vi "NML data acq file names extract.vi"(0 "assign directory":bool, 1 "File name header":string="BaCrO_CCR", 3 "path in":path, 5 "From":string="12\n", 7 "To":string="2", 9 "Excluding From":string, 11 "Excluding To":string) -> (4 "path out":path, 6 "file paths":string[](array[string]), 10 "filtered  numbers":string[](array[string])=["002", "003", "004", "005", "006", "007", "008", "009", "010", "011", "012"], 15 "existing files":string[](array[string]))   [LabVIEW 2019]
panel:
  in  "File name extension":string=".txt"
  # "The new version of NML Data Acq adds extension \"txt\". \nThe program will try to identify  which\n version was used."
  # "."
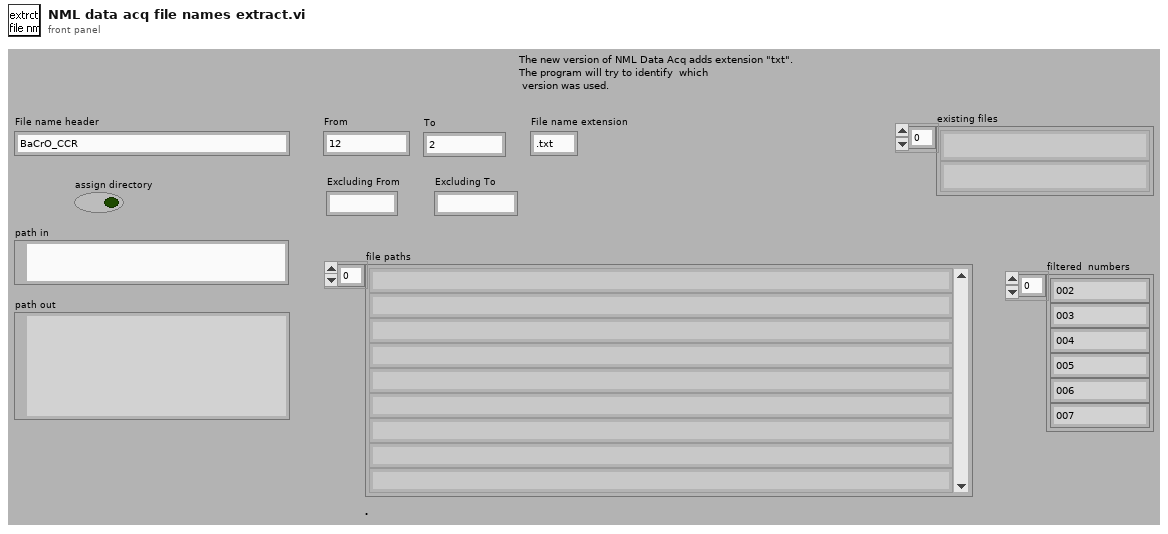
[diagram p1: front panel]
types:
  T1 = enum32{"existing file", "new file", "new or existing file", "existing dir", "new dir", "new or existing dir", "existing file (use LLBs)", "new file (use LLBs)", "new or existing file (use LLBs)", "new or existing file or directory (use LLBs)"}
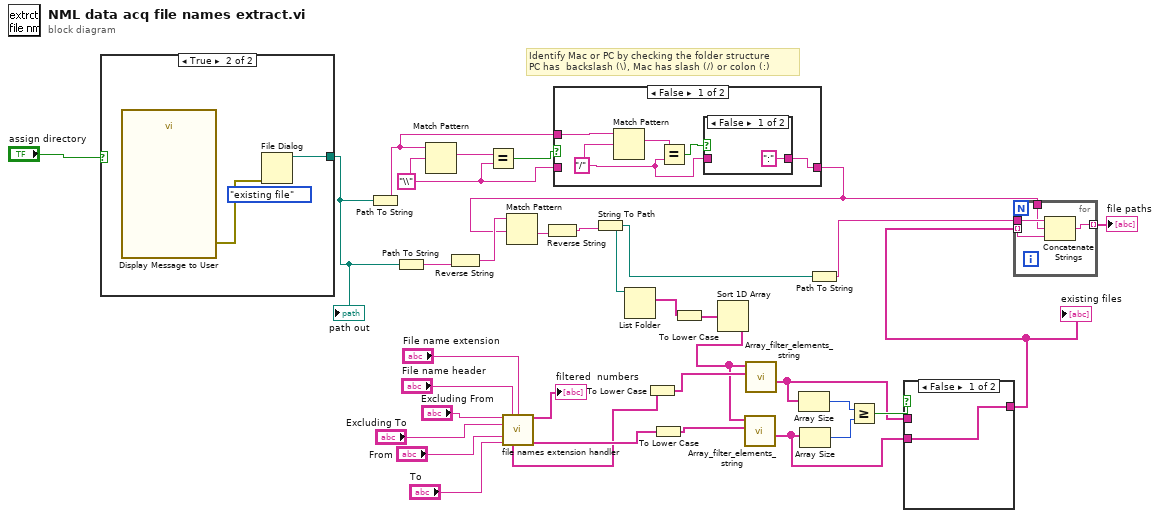
[diagram p0: block diagram]
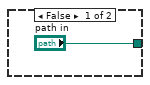
[diagram p3: hidden frame]
diagram:
  w25 = "\\" ("regular expression")
  # "Identify Mac or PC by checking the folder structure\nPC has  backslash (\\), Mac has slash (/) or colon (:)"
  n1 = case shown="True" "assign directory" {
    tunnel: ["path in" w37] -> w23
    frame False {
    }
    frame True {
      (unwired) T1."existing file" ("select mode (2)")
      n2 = call "Display Message to User"() -> ("error out"=w36:errorcluster)  [unwired: 10 in, 1 out]
      n3 = File Dialog(8:w36) -> (3:w37:path)  [unwired: 9 out]
    }
  }
  "path out" <- w23
  n4 = Path To String(path=w23) -> (string=w18:string)
  n5 = Path To String(path=w23) -> (string=w34:string)
  n6 = Match Pattern(string=w18, regular expression=w25) -> (match substring=w27:string)  [unwired: 4 out]
  n7 = Reverse String(1:w34) -> (0:w33:string)
  n8 = Equal?(x=w27, y=w25) -> (x = y?=w26:bool)
  n9 = call "file names extension handler.vi"("exclude1"="Excluding From", "File name header"="File name header", "File name extension"="File name extension", "exclude2"="Excluding To", "include 1"="From", "include 2"="To") -> ("filtered  numbers"=→"filtered  numbers":string[], "filetered file names"=w8:string[], "filtered file name no ext"=w9:string[])  [unwired: 6 in, 1 out]
  n10 = case shown="False" w26 {
    tunnel: [w39 w45] -> w19
    tunnel: w25 -> [_ w45]
    tunnel: w18 -> [w42 _]
    frame False {
      w38 = "/" ("regular expression")
      n11 = Match Pattern(string=w42, regular expression=w38) -> (match substring=w41:string)  [unwired: 4 out]
      n12 = Equal?(x=w41, y=w38) -> (x = y?=w40:bool)
      n13 = case shown="False" w40 {
        tunnel: [":" ("regular expression") w44] -> w39
        tunnel: w38 -> [_ w44]
        frame False {
        }
        frame True {
        }
      }
    }
    frame True {
    }
  }
  n14 = Match Pattern(string=w33, regular expression=w19) -> (after substring=w31:string)  [unwired: 4 out]
  n15 = Reverse String(1:w31) -> (0:w32:string)
  n16 = String To Path(string=w32) -> (path=w30:path)
  n17 = List Folder(path=w30) -> (filenames=w28:string[])  [unwired: 1 in, 5 out]
  n18 = To Lower Case(string=w8) -> (all lower case string=w22:string[])
  n19 = To Lower Case(string=w9) -> (all lower case string=w10:string[])
  n20 = To Lower Case(string=w28) -> (all lower case string=w29:string[])
  n21 = Sort 1D Array(array=w29) -> (sorted array=w11:string[])
  n22 = call "Array_filter_elements_string.vi"("set2"=w10, "set1"=w11) -> ("shared"=w3:string[])  [unwired: 7 in, 2 out]
  n23 = call "Array_filter_elements_string.vi"("set2"=w22, "set1"=w11) -> ("shared"=w4:string[])  [unwired: 7 in, 2 out]
  n24 = Array Size(array=w4) -> (size(s)=w7:i32)
  n25 = Array Size(array=w3) -> (size(s)=w6:i32)
  n26 = Path To String(path=w30) -> (string=w21:string)
  n27 = Greater Or Equal?(x=w7, y=w6) -> (x >= y?=w5:bool)
  n28 = case shown="False" w5 {
    tunnel: [w46 w47] -> w2
    tunnel: w4 -> [_ w47]
    tunnel: w3 -> [w46 _]
    frame False {
    }
    frame True {
    }
  }
  "existing files" <- w2
  n29 = for {
    tunnel: w21 -> [w51]
    tunnel: w2 -> [w49] mode=indexing
    tunnel: [w50] -> w20 mode=indexing
    tunnel: w19 -> [w48]
    n30 = Concatenate Strings(w51, w48, w49) -> (w50:string)
  }
  "file paths" <- w20
